vi "Init Task.vi"(4 "counter":tag, 6 "line grouping":i32(ring) items=["one channel for each line", "one channel for all lines"], 7 "physical channels":tag, 8 "error in (no error)":errorcluster, 9 "name":string, 10 "DAQmxTaksContainer_General IN":refnum<class "DAQmxTaksContainer_General.lvclass">, 11 "DAQmxTaskAITension_Emulate in":refnum<class "DAQmxTaskAIVoltage_Emulate.lvclass">) -> (0 "error out":errorcluster, 3 "DAQmxTaskAITension_Emulate out":refnum<class "DAQmxTaskAIVoltage_Emulate.lvclass">)   [LabVIEW 2015, in "DAQmxTaskAIVoltage_Emulate.lvclass"]
uses:
  DAQmxTaskAIVoltage_Emulate.lvclass
  DAQmxTaskContainer_General/DAQmxTaksContainer_General.lvclass
  DAQmxTask.lvclass/DAQmxTask.ctl
  DAQmxTask.lvclass
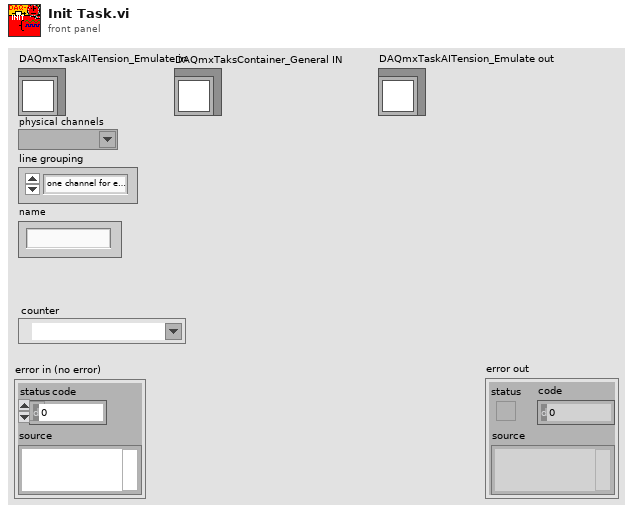
[diagram p1: front panel]
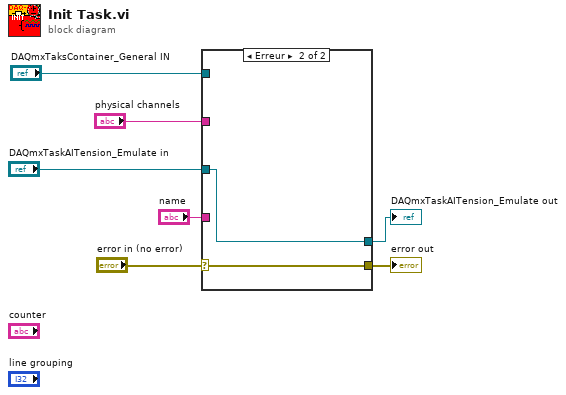
[diagram p0: block diagram]
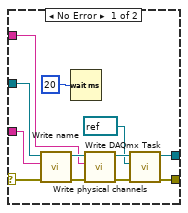
[diagram p2: hidden frame]
diagram:
  n1 = case shown="Erreur" "error in (no error)" {
    selector: "error in (no error)" -> [w15 w21]
    tunnel: "DAQmxTaskAITension_Emulate in" -> [w16 w20]
    tunnel: "name" -> [w10 _]
    tunnel: [w8 w21] -> w4
    tunnel: "physical channels" -> [w13 _]
    tunnel: "DAQmxTaksContainer_General IN" -> [_ _]
    tunnel: [w9 w20] -> w1
    frame No Error {
      n2 = call "Write name.vi"("error in (no error)"=w15, "name"=w10, "DAQmxTask in"=w16) -> ("error out"=w19:errorcluster, "DAQmxTask out"=w18:refnum<class "DAQmxTaskAIVoltage_Emulate.lvclass">)  [unwired: 7 in]
      n3 = Wait (ms)(milliseconds to wait=u32 20) -> ()  [unwired: 1 out]
      n4 = call "Write physical channels.vi"("error in (no error)"=w19, "physical channels"=w13, "DAQmxTask in"=w18) -> ("error out"=w14:errorcluster, "DAQmxTask out"=w17:refnum<class "DAQmxTaskAIVoltage_Emulate.lvclass">)  [unwired: 7 in]
      n5 = call "Write DAQmx Task.vi"("error in (no error)"=w14, "DAQmx Task Name"=refnum<k21> refnum, "DAQmxTask in"=w17) -> ("error out"=w8:errorcluster, "DAQmxTask out"=w9:refnum<class "DAQmxTaskAIVoltage_Emulate.lvclass">)  [unwired: 7 in]
    }
    frame Error {
    }
  }
  "error out" <- w4
  "DAQmxTaskAITension_Emulate out" <- w1
